vi "FB Switch Output Error.vi"(8 "error in":errorcluster) -> (0 "error out":errorcluster)   [LabVIEW 2017]
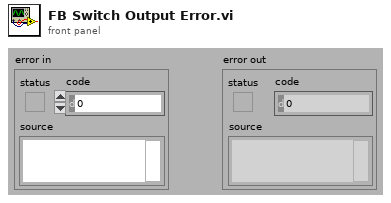
[diagram p1: front panel]
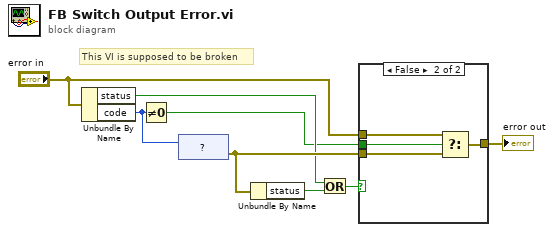
[diagram p0: block diagram]
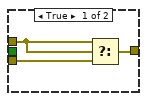
[diagram p2: hidden frame]
diagram:
  # "This VI is supposed to be broken"
  n1 = Unbundle By Name("error in") -> ("status"=w4:bool, "code"=w1:i32)
  n2 = Not Equal To 0?(x=w1) -> (x != 0?=w2:bool)
  n3 = shared-variable "?"(w1) -> (error out=w6:errorcluster)  [unwired: 1 in]
  n4 = Unbundle By Name(w6) -> ("status"=w5:bool)
  n5 = Or(x=w4, y=w5) -> (x .or. y?=w3:bool)
  n6 = case shown="False" w3 {
    tunnel: "error in" -> [w9 w13]
    tunnel: [w11 w15] -> w7
    tunnel: w6 -> [w10 w14]
    tunnel: w2 -> [_ w12]
    frame True {
      n7 = Select(t=w9, s=w9, f=w10) -> (s? t:f=w11:errorcluster)
    }
    frame False {
      n8 = Select(t=w13, s=w12, f=w14) -> (s? t:f=w15:errorcluster)
    }
  }
  "error out" <- w7
